vi "testRPM.vi"() -> ()   [LabVIEW 2014]
uses:
  <vilib>/Analysis/baseanly.llb/Mean (DBL).vi
  <vilib>/Analysis/NI_AALBase.lvlib
panel:
  out "Filtered Signal 2":dynamicdata(graph) caption="Filtered Signal"
  out "error out":errorcluster
  in  "stop":bool
  in  "Frequency 2":dbl=10.1 caption="Frequency"
  out "Frequency":dbl
  out "Filtered Signal":dynamicdata(graph)
  out "Sawtooth with Gaussian Noise":dynamicdata(graph)
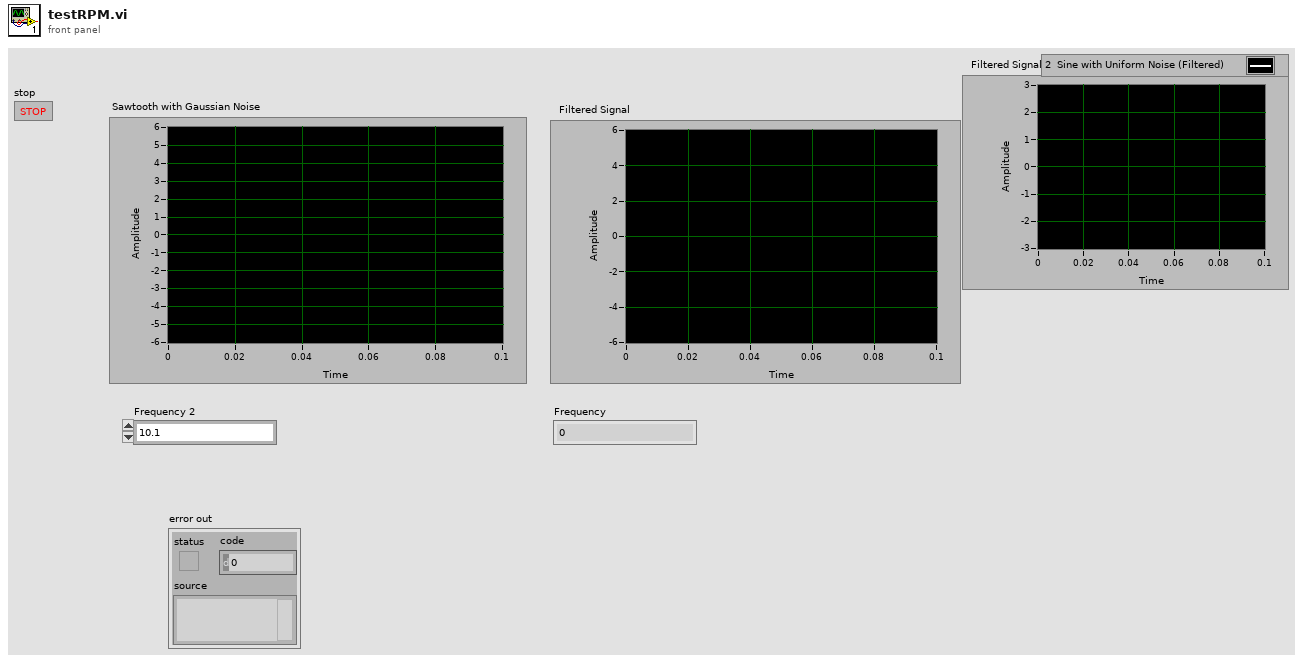
[diagram p1: front panel]
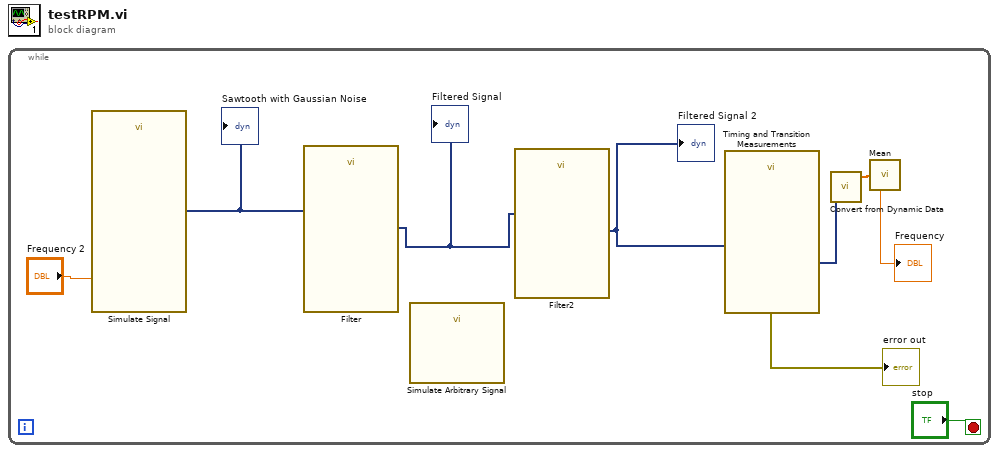
[diagram p0: block diagram]
diagram:
  n1 = while {
    stop <- "stop" stop-if-true
    n2 = call "Simulate Signal"("Frequency"="Frequency 2") -> ("Sine with Uniform Noise"=w9:dynamicdata)  [unwired: 13 in, 1 out]
    "Sawtooth with Gaussian Noise" <- w9
    n3 = call "Filter"("Signal"=w9) -> ("Filtered Signal"=w5:dynamicdata)  [unwired: 9 in, 1 out]
    "Filtered Signal" <- w5
    n4 = call "Simulate Arbitrary Signal"() -> ()  [unwired: 9 in, 3 out]
    n5 = call "Filter2"("Signal"=w5) -> ("Filtered Signal"=w4:dynamicdata)  [unwired: 9 in, 1 out]
    "Filtered Signal 2" <- w4
    n6 = call "Timing and Transition Measurements"("Signals"=w4) -> ("error out"=→"error out":errorcluster, "Frequency"=w3:dynamicdata)  [unwired: 9 in]
    n7 = call "Convert from Dynamic Data"("Dynamic Data Type"=w3) -> ("Array"=w2:dbl[])  [unwired: 3 in]
    n8 = call-poly <vilib>:"Mean.vi"("X"=w2) -> ("mean"=→"Frequency":dbl)  [unwired: 1 out]
  }
